vi "Get Named Item From Namespaced Element.vi"(6 "Tag":string, 8 "error in (no error)":errorcluster, 9 "Local Name":string, 10 "Namespace URI":string, 11 "DOM document in":refnum<k20>) -> (0 "error out":errorcluster, 2 "Value":string, 3 "DOM document out":refnum<k20>)   [LabVIEW 2012]
uses:
  <vilib>/xml/Close Reference(Node).vi
  <vilib>/xml/Close Reference(NNMap).vi
  <resource>/objmgr/DOMUserDefRef.rc
  <vilib>/xml/NI_XML.lvlib
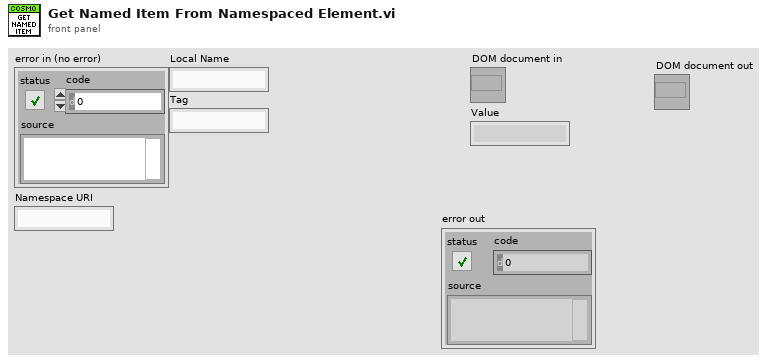
[diagram p1: front panel]
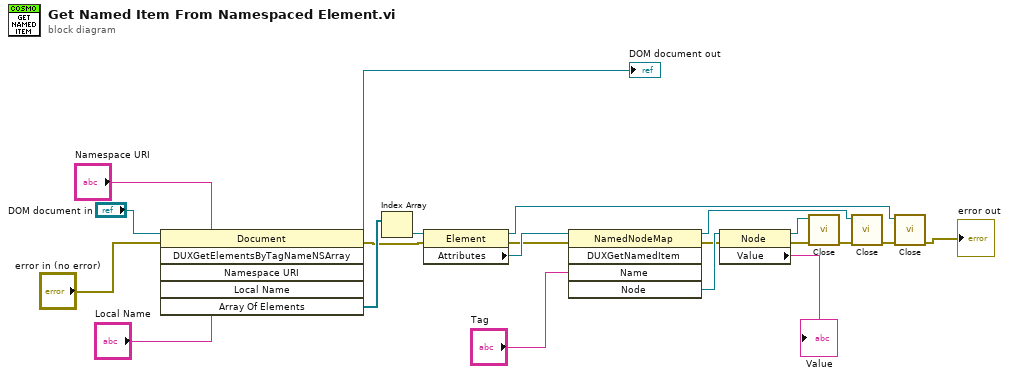
[diagram p0: block diagram]
diagram:
  n1 = invoke class="Document" method="DUXGetElementsByTagNameNSArray"(reference="DOM document in", error in="error in (no error)", "Namespace URI"="Namespace URI", "Local Name"="Local Name") -> (reference out=→"DOM document out":refnum<k20>, error out=w7:errorcluster, "Array Of Elements"=w21:refnum<k20>[])  [unwired: 2 in, 3 out]
  n2 = Index Array(array=w21) -> (element=w20:refnum<k20>)  [unwired: 1 in]
  n3 = property class="Element"(reference=w20, error in=w7) -> (reference out=w10:refnum<k20>, error out=w18:errorcluster, "Attributes"=w19:refnum<k20>)
  n4 = invoke class="NamedNodeMap" method="DUXGetNamedItem"(reference=w19, error in=w18, "Name"="Tag") -> (reference out=w12:refnum<k20>, error out=w16:errorcluster, "Node"=w17:refnum<k20>)  [unwired: 2 in, 2 out]
  n5 = property class="Node"(reference=w17, error in=w16) -> (reference out=w15:refnum<k20>, error out=w14:errorcluster, "Value"=→"Value":string)
  n6 = call-poly <vilib>:"Close.vi"("error in (no error)"=w14, "node"=w15) -> ("error out"=w13:errorcluster)  [unwired: 7 in]
  n7 = call-poly <vilib>:"Close.vi"("error in (no error)"=w13, "named node map"=w12) -> ("error out"=w11:errorcluster)  [unwired: 7 in]
  n8 = call-poly <vilib>:"Close.vi"("error in (no error)"=w11, "node"=w10) -> ("error out"=→"error out":errorcluster)  [unwired: 7 in]
